vi "sub_RN16reader.vi"(11 "Bit Sequence":i16[](array[numeric])) -> (3 "Bits RN16":i16[](array[numeric]))   [LabVIEW 2015]
panel:
  out "length":i32
  out "text":string
  in  "Path":path
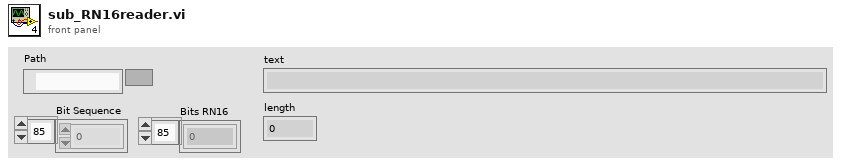
[diagram p1: front panel]
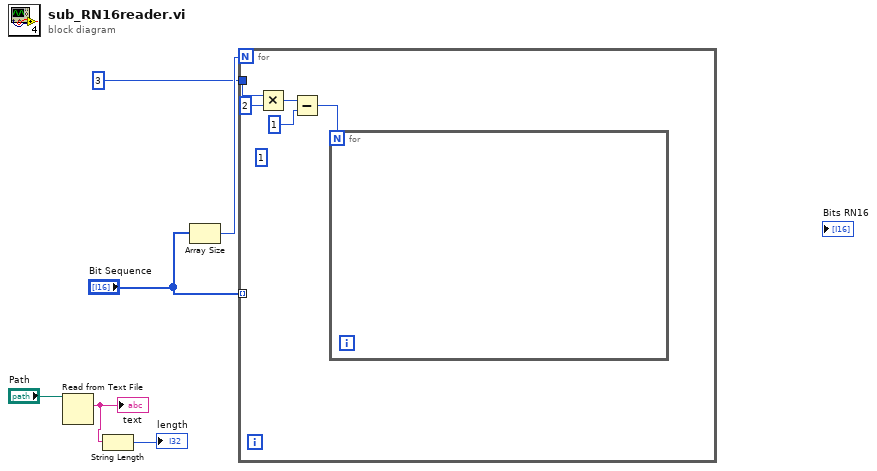
[diagram p0: block diagram]
diagram:
  n1 = Read from Text File(file (use dialog)="Path") -> (text=w2:string)  [unwired: 3 in, 3 out]
  "text" <- w2
  n2 = String Length(string=w2) -> (length=→"length":i32)
  n3 = Array Size(array="Bit Sequence") -> (size(s)=w6:i32)
  n4 = for {
    N: w6 -> [_]
    tunnel: "Bit Sequence" -> [_] mode=indexing
    tunnel: 3 -> [w11]
    (unwired) 1
    n5 = Multiply(x=w11, y=2) -> (x*y=w9:i32)
    n6 = Subtract(x=w9, y=1) -> (x-y=w7:i32)
    n7 = for {
      N: w7 -> [_]
    }
  }
